vi "setMeasurements.vi"(7 "Pressure":dbl, 8 "error in (no error)":errorcluster, 9 "Humidity":dbl, 10 "Temperature":dbl, 11 "WeatherData.lvclass":refnum<class "WeatherData.lvclass">) -> (0 "error out":errorcluster, 3 "WeatherData.lvclass 2":refnum<class "WeatherData.lvclass">)   [LabVIEW 2020, in "WeatherData.lvclass"]
uses:
  WeatherData.lvclass
  WeatherData.lvclass/WeatherData.ctl
panel:
  # "Connector Pane"
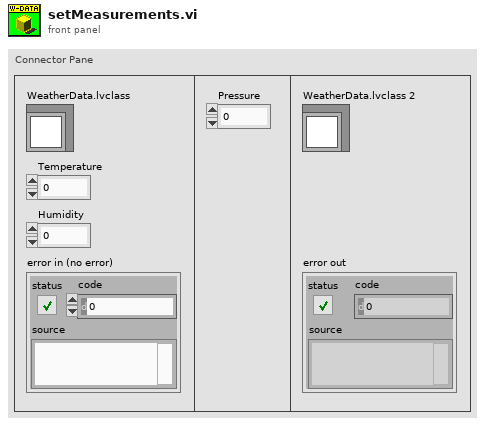
[diagram p1: front panel]
types:
  T1 = typedef "weatherDataCluster.ctl" = cluster{"Temperature":dbl, "Humidity":dbl, "Pressure":dbl, "Observers":refnum<class "Observer.lvclass">[]}
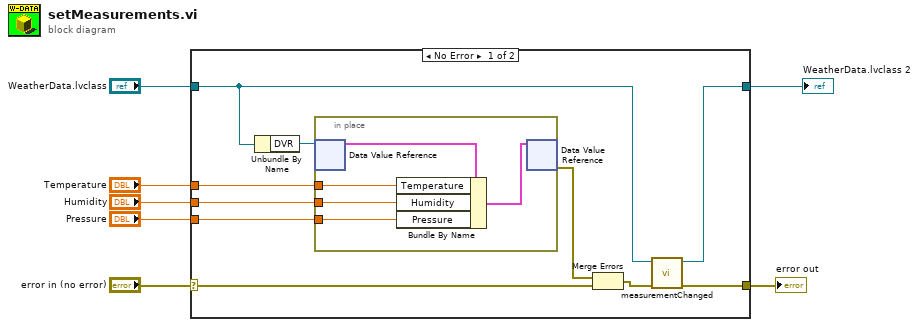
[diagram p0: block diagram]
diagram:
  n1 = case shown="No Error" "error in (no error)" {
    selector: "error in (no error)" -> [w17 w23]
    tunnel: [w16 w23] -> w6
    tunnel: [w15 w24] -> w5
    tunnel: "Temperature" -> [w13 _]
    tunnel: "Humidity" -> [w12 _]
    tunnel: "Pressure" -> [w11 _]
    tunnel: "WeatherData.lvclass" -> [w8 w24]
    frame No Error {
      n2 = Unbundle By Name(w8) -> ("DVR"=w14:refnum<data-value>)
      n3 = in-place {
        in-place-border: w13 -> [w20]
        in-place-border: w12 -> [w19]
        in-place-border: w11 -> [w18]
        n4 = in-place-dvr #1(w14) -> (w22:T1)  [unwired: 1 out]
        n5 = Bundle By Name(cluster=w22, "Temperature"=w20, "Humidity"=w19, "Pressure"=w18) -> (w21:T1)
        n6 = in-place-dvr #1(w21) -> (w9:errorcluster)  [unwired: 1 out]
      }
      n7 = Merge Errors(w9, w17) -> (w10:errorcluster)
      n8 = call "measurementChanged.vi"("error in (no error)"=w10, "WeatherData.lvclass"=w8) -> ("error out"=w16:errorcluster, "WeatherData.lvclass 2"=w15:refnum<class "WeatherData.lvclass">)  [unwired: 8 in]
    }
    frame Error {
    }
  }
  "WeatherData.lvclass 2" <- w5
  "error out" <- w6
